vi "BRig_Host_dataRunState_dataTS_tSelection_plot.vi"() -> (2 "output_idx_dataTS_tSelection_plot":i32)   [LabVIEW 2014]
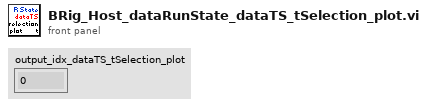
[diagram p1: front panel]
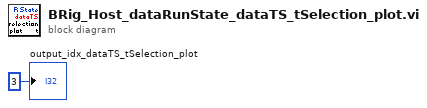
[diagram p0: block diagram]
diagram:
  "output_idx_dataTS_tSelection_plot" <- 3 ("output_idx_dataTS")
